vi "Get (String 2D Array).vi"(5 "Tag":string, 7 "error in (no error)":errorcluster, 10 "ByRef Variant Repsitory in":refnum<data-value>) -> (0 "error out":errorcluster, 3 "Values":string[][](array[string]))   [LabVIEW 2015, in "ByRef Variant Repository.lvlib"]
uses:
  ByRef Variant Repository.lvlib
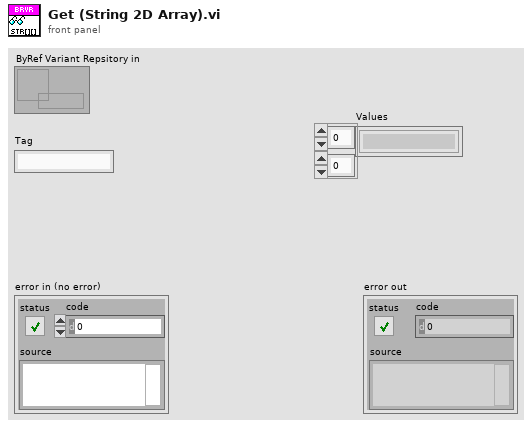
[diagram p1: front panel]
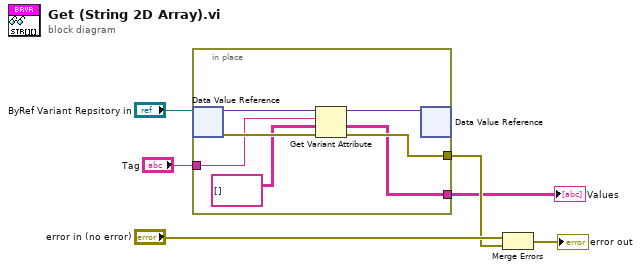
[diagram p0: block diagram]
diagram:
  n1 = in-place {
    in-place-border: [w10] -> w4
    in-place-border: "Tag" -> [w9]
    in-place-border: [w8] -> w2
    n2 = in-place-dvr #1("ByRef Variant Repsitory in") -> (w12:variant, w13:errorcluster)
    n3 = Get Variant Attribute(Variant=w12, name=w9, default value (empty Variant)=string[][] [], error in=w13) -> (duplicate Variant=w11:variant, value=w8:string[][], error out=w10:errorcluster)  [unwired: 1 out]
    n4 = in-place-dvr #1(w11) -> ()  [unwired: 2 out]
  }
  "Values" <- w2
  n5 = Merge Errors("error in (no error)", w4) -> (→"error out":errorcluster)
